vi "J-eV.vi"(2 "eV":dbl, 3 "J":dbl) -> (0 "J":dbl, 1 "eV":dbl)   [LabVIEW 2019]
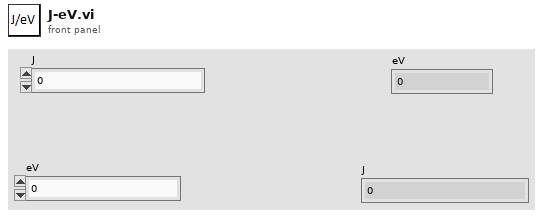
[diagram p1: front panel]
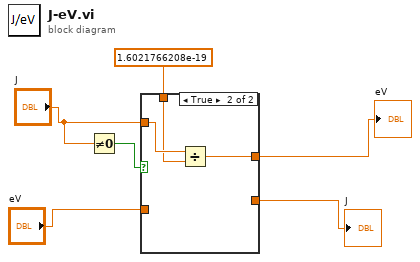
[diagram p0: block diagram]
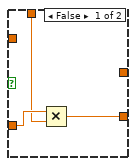
[diagram p2: hidden frame]
diagram:
  n1 = Not Equal To 0?(x="J") -> (x != 0?=w6:bool)
  n2 = case shown="True" w6 {
    tunnel: "J" -> [_ w12]
    tunnel: 1.6021766208e-19 -> [w8 w11]
    tunnel: [_ w10] -> w4
    tunnel: "eV" -> [w9 _]
    tunnel: [w7 _] -> w2
    frame False {
      n3 = Multiply(x=w9, y=w8) -> (x*y=w7:dbl)
    }
    frame True {
      n4 = Divide(x=w12, y=w11) -> (x/y=w10:dbl)
    }
  }
  "eV" <- w4
  "J" <- w2
